vi "CRYCheck EditVal.vi"(8 "Is SubPan?":bool, 9 "display message?":bool, 10 "Flatten Element":string, 11 "MCListbox Refnum":refnum<vi>) -> (3 "Error":bool)   [LabVIEW 2013]
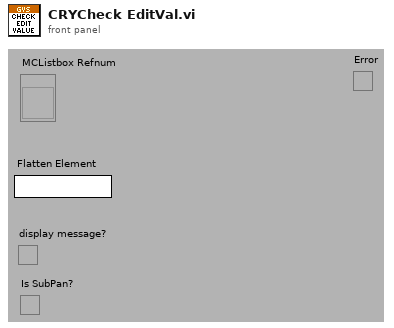
[diagram p1: front panel]
types:
  T1 = typedef "CRYStimulus Parameter.ctl" = cluster{"Name":string, "Level Out":dbl, "Start Freq":dbl, "Stop Freq":dbl, "Steps":u32, "Cycles":u32, "Sweep type":i32, "Freq":dbl, "Start ampl":dbl, "Stop ampl":dbl, "sine waves":cluster{"freq":dbl, "ampl":dbl, "cycles":dbl}[], "wav path":string, "Sweep time":dbl, "Resolution":u16, "Tone type6":u16, "fix/ratio6":u16, "Ratio6":u16, "Difference6":u32, "RatioFreq6":u32}
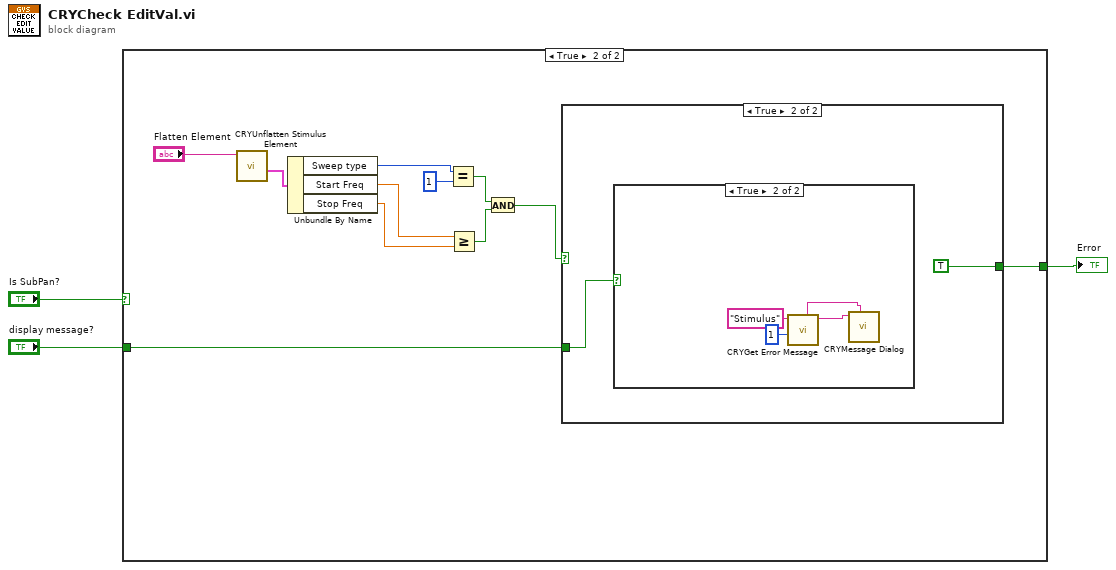
[diagram p0: block diagram]
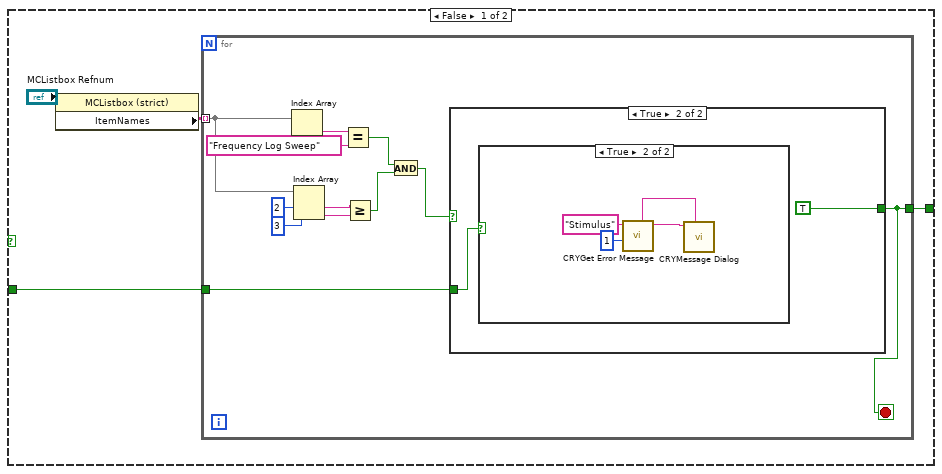
[diagram p2: hidden frame]
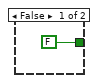
[diagram p3: hidden frame]
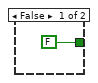
[diagram p5: hidden frame]
diagram:
  n1 = case shown="True" "Is SubPan?" {
    tunnel: "display message?" -> [w5 w28]
    tunnel: [w4 w27] -> w1
    frame False {
      n2 = property class="MCListbox (strict)"(reference="MCListbox Refnum") -> ("ItemNames"=w6:string[][])  [unwired: 1 in, 2 out]
      n3 = for {
        tunnel: w6 -> [w17] mode=indexing
        tunnel: w5 -> [w9]
        tunnel: [w8] -> w4
        stop <- w8 stop-if-true
        n4 = Index Array(array=w17) -> (element=w19:string)  [unwired: 1 in]
        n5 = Index Array(array=w17, index #1=2 ("index"), index #2=3 ("index")) -> (element #1=w13:string, element #2=w14:string)
        n6 = Equal?(x=w19, y="Frequency Log Sweep") -> (x = y?=w12:bool)
        n7 = Greater Or Equal?(x=w13, y=w14) -> (x >= y?=w11:bool)
        n8 = And(x=w12, y=w11) -> (x .and. y?=w10:bool)
        n9 = case shown="True" w10 {
          tunnel: w9 -> [_ w22]
          tunnel: [FALSE ("Error") TRUE ("Error")] -> w8
          frame False {
          }
          frame True {
            n10 = case shown="True" w22 {
              frame False {
              }
              frame True {
                n11 = call "CRYGet Error Message.vi"("Error No"=1, "Kind"="Stimulus") -> ("Message"=w24:string, "Window Title"=w23:string)  [unwired: 4 in, 4 out]
                n12 = call "CRYMessage Dialog.vi"("Window Title"=w23, "Message Content"=w24) -> ()  [unwired: 8 in, 2 out]
              }
            }
          }
        }
      }
    }
    frame True {
      n13 = call "CRYUnflatten Stimulus Element.vi"("Unflatten Stimulus Element setup"="Flatten Element") -> ("Stimulus Para"=w36:T1)  [unwired: 1 in, 9 out]
      n14 = Unbundle By Name(w36) -> ("Sweep type"=w35:i32, "Start Freq"=w33:dbl, "Stop Freq"=w32:dbl)
      n15 = Equal?(x=w35, y=1) -> (x = y?=w31:bool)
      n16 = Greater Or Equal?(x=w33, y=w32) -> (x >= y?=w30:bool)
      n17 = And(x=w31, y=w30) -> (x .and. y?=w29:bool)
      n18 = case shown="True" w29 {
        tunnel: w28 -> [_ w40]
        tunnel: [FALSE ("Error") TRUE ("Error")] -> w27
        frame False {
        }
        frame True {
          n19 = case shown="True" w40 {
            frame False {
            }
            frame True {
              n20 = call "CRYGet Error Message.vi"("Error No"=1, "Kind"="Stimulus") -> ("Message"=w42:string, "Window Title"=w41:string)  [unwired: 4 in, 4 out]
              n21 = call "CRYMessage Dialog.vi"("Window Title"=w41, "Message Content"=w42) -> ()  [unwired: 8 in, 2 out]
            }
          }
        }
      }
    }
  }
  "Error" <- w1
